vi "OpenVS.vi"(11 "Visible?":bool) -> ()   [LabVIEW 2015, in "MiscHelperVIs.lvlib"]
uses:
  MiscHelperVIs.lvlib
  <vilib>/Utility/sysdir.llb/System Directory Type.ctl
panel:
  # "This VI calls VS silently if passed a True"
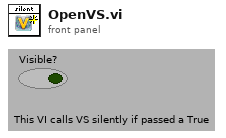
[diagram p1: front panel]
types:
  T1 = typedef "System Directory Type.ctl" = i32
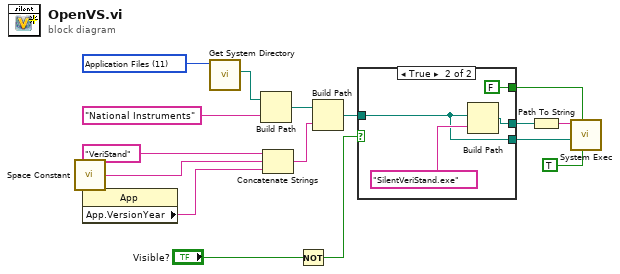
[diagram p0: block diagram]
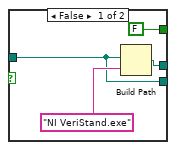
[diagram p2: hidden frame]
diagram:
  w15 = T1 11 items=["User Home"=0, "User Desktop"=1, "User Documents"=2, "User Application Data"=3, "User Preferences"=4, "User Temporary"=5, "Public Documents"=6, "Public Application Data"=7, "Public Preferences"=8, "Public Cache"=13, "System Core Libraries"=9, "System Installed Libraries"=10, "Application Files"=11, "Boot Volume Root"=12] ("system directory type")
  n1 = call <vilib>:"Space Constant.vi"() -> ("String"=w6:string)
  n2 = property class="App"() -> ("App.VersionYear"=w7:string)  [unwired: 2 in, 2 out]
  n3 = call <vilib>:"Get System Directory.vi"("system directory type"=w15) -> ("system directory"=w14:path)  [unwired: 10 in]
  n4 = Build Path(base path=w14, name or relative path="National Instruments") -> (appended path=w12:path)
  n5 = Concatenate Strings("VeriStand" ("name or relative path"), w6, w7) -> (w5:string)
  n6 = Not(x="Visible?") -> (.not. x?=w1:bool)
  n7 = Build Path(base path=w12, name or relative path=w5) -> (appended path=w9:path)
  n8 = case shown="True" w1 {
    tunnel: [w19 w23] -> w11
    tunnel: w9 -> [w18 w22]
    tunnel: [w18 w22] -> w4
    tunnel: [FALSE ("wait until completion? (T)") FALSE ("wait until completion? (T)")] -> w3
    frame False {
      n9 = Build Path(base path=w18, name or relative path="NI VeriStand.exe") -> (appended path=w19:path)
    }
    frame True {
      n10 = Build Path(base path=w22, name or relative path="SilentVeriStand.exe") -> (appended path=w23:path)
    }
  }
  n11 = Path To String(path=w11) -> (string=w10:string)
  n12 = call <vilib>:"System Exec.vi"("run minimized? (F)"=TRUE, "wait until completion? (T)"=w3, "working directory"=w4, "command line"=w10) -> ()  [unwired: 4 in, 4 out]
